vi "checkin.vi"(8 "error in (no error)":errorcluster, 11 "GenericImageAssembler in":refnum<class "GenericImageAssembler.lvclass">) -> (0 "error out":errorcluster, 3 "GenericImageAssembler out":refnum<class "GenericImageAssembler.lvclass">)   [LabVIEW 2010, in "GenericImageAssembler.lvclass"]
uses:
  GenericImageAssembler.lvclass
  common/classes/GenericToplevelComponent/GenericToplevelComponent/GenericToplevelComponent.lvclass
  class_data.vi
  common/classes/GenericComponent/GenericComponent/GenericComponent.lvclass
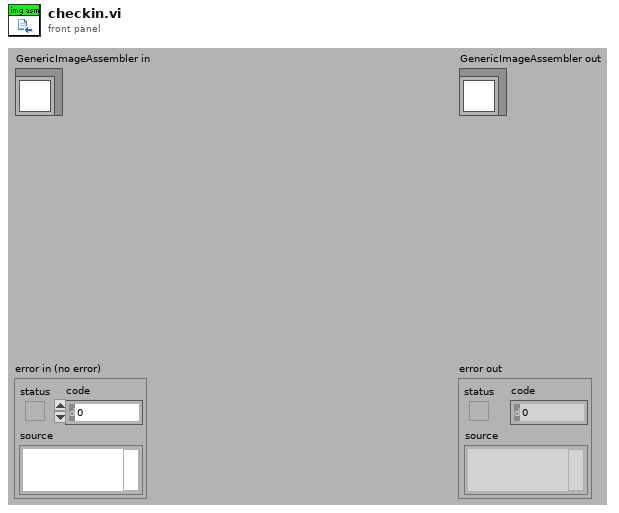
[diagram p1: front panel]
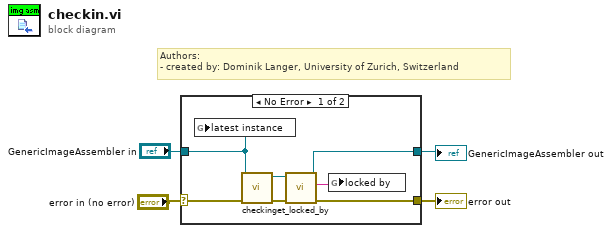
[diagram p0: block diagram]
diagram:
  # "Authors: \n- created by: Dominik Langer, University of Zurich, Switzerland"
  n1 = case shown="No Error" "error in (no error)" {
    selector: "error in (no error)" -> [w8 w13]
    tunnel: [w11 w13] -> w3
    tunnel: [w9 w12] -> w4
    tunnel: "GenericImageAssembler in" -> [w7 w12]
    frame No Error {
      n2 = global write "class_data.vi" "latest instance"(w7) -> ()
      n3 = call-parent "checkin.vi"("error in (no error)"=w8, "GenericPlugin in"=w7) -> ("error out"=w5:errorcluster, "GenericPlugin out"=w6:refnum<class "GenericImageAssembler.lvclass">)  [unwired: 8 in]
      n4 = call "get_locked_by.vi"("error in (no error)"=w5, "GenericPlugin.lvclass in"=w6) -> ("error out"=w11:errorcluster, "locked by"=w10:string, "GenericPlugin.lvclass out"=w9:refnum<class "GenericImageAssembler.lvclass">)  [unwired: 7 out]
      n5 = global write "class_data.vi" "locked by"(w10) -> ()
    }
    frame Error {
    }
  }
  "error out" <- w3
  "GenericImageAssembler out" <- w4
